vi "Auto Control.vi"   [LabVIEW 2018]
uses:
  <vilib>/Rock Robotics/Network Tables/NT Write String Array.vi
  SubSystems/Drive Train/Drive Train Global.vi
  Robot Global Data.vi
  SubSystems/Hatch Panel Intake/Hatch Panel Intake Global.vi
  SubSystems/Lift/Lift Global.vi
  SubSystems/Cargo Intake/Cargo Intake Global.vi
types:
  T1 = cluster{"X PID":cluster{"proportional gain (Kc)":dbl, "integral time (Ti, min)":dbl, "derivative time (Td, min)":dbl}, "Y PID":cluster{"proportional gain (Kc)":dbl, "integral time (Ti, min)":dbl, "derivative time (Td, min)":dbl}, "Z PID":cluster{"proportional gain (Kc)":dbl, "integral time (Ti, min)":dbl, "derivative time (Td, min)":dbl}}
  T2 = enum16{"Hatch Panel Zone 1", "Hatch Panel Zone 2", "Hatch Panel Zone 3", "Cargo Zone 1", "Cargo Zone 2", "Cargo Zone 3", "Cargo Ship Zone"}
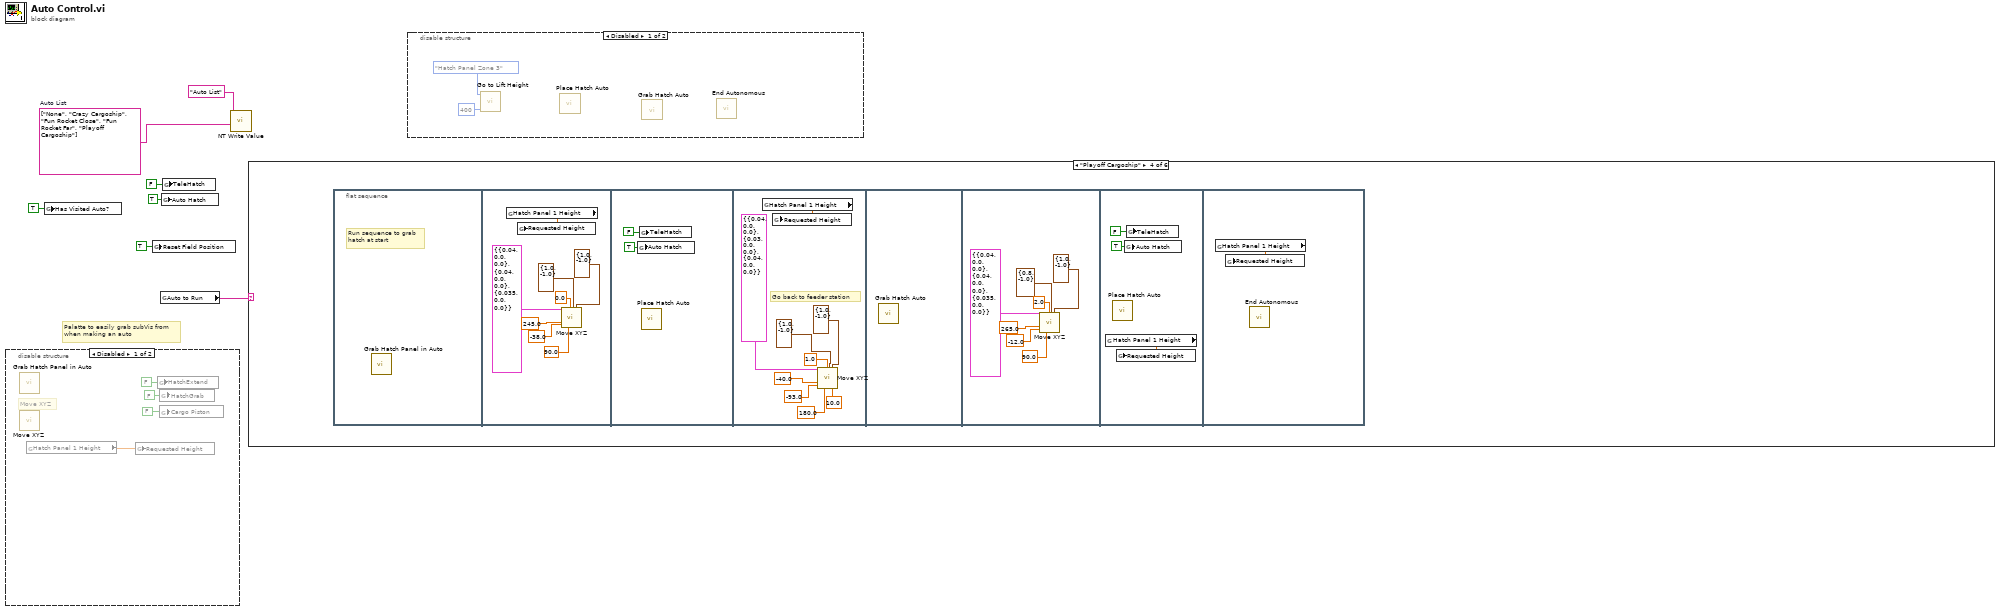
[diagram p0: block diagram]
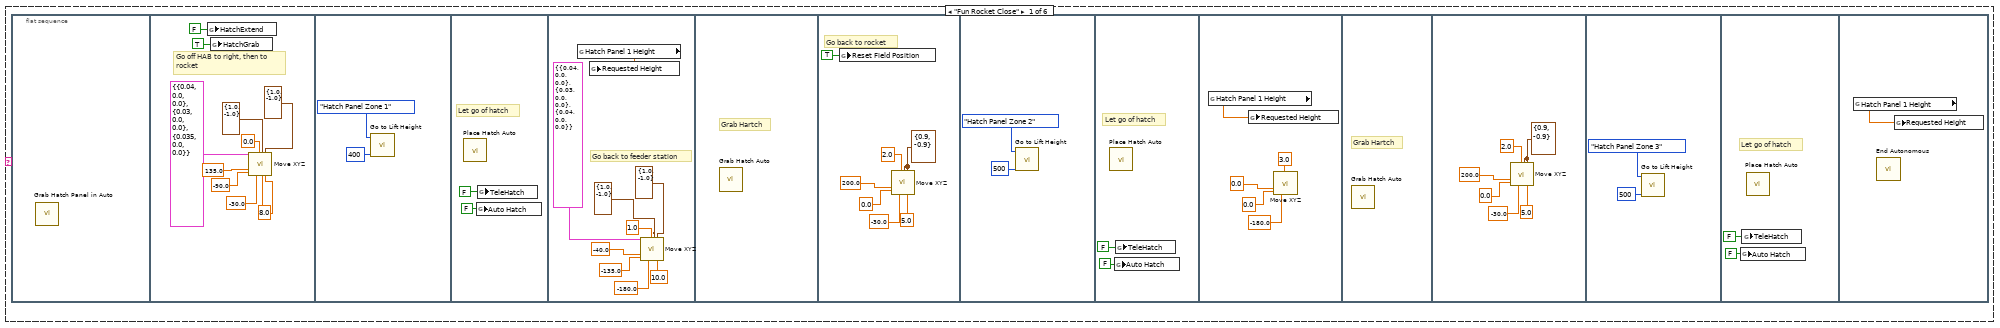
[diagram p4: hidden frame]
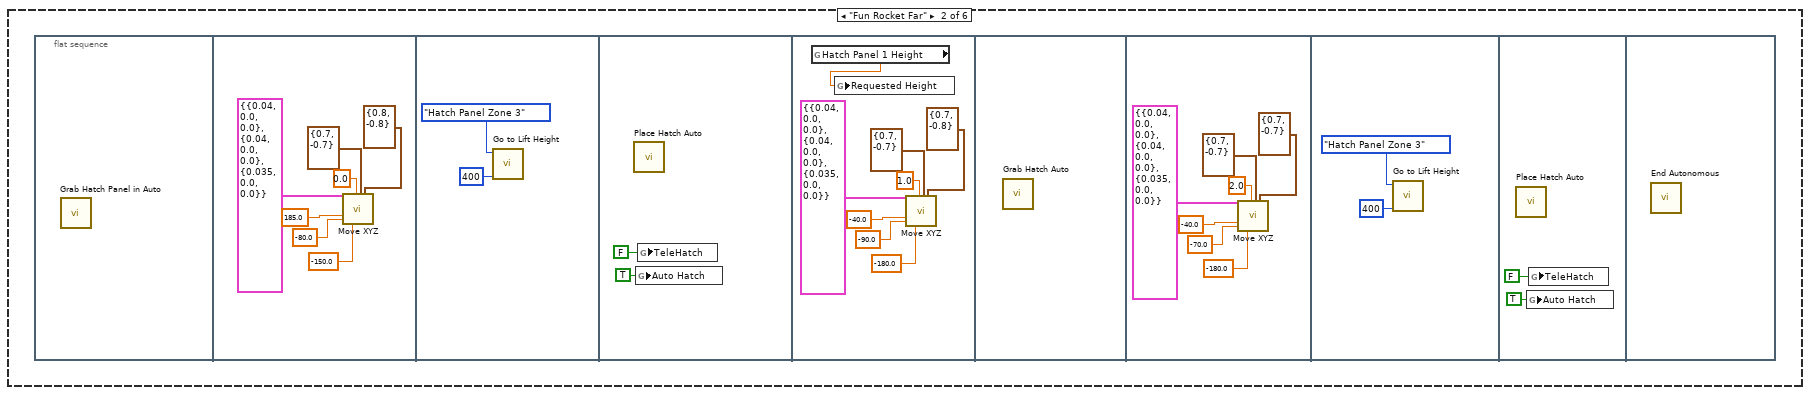
[diagram p5: hidden frame]
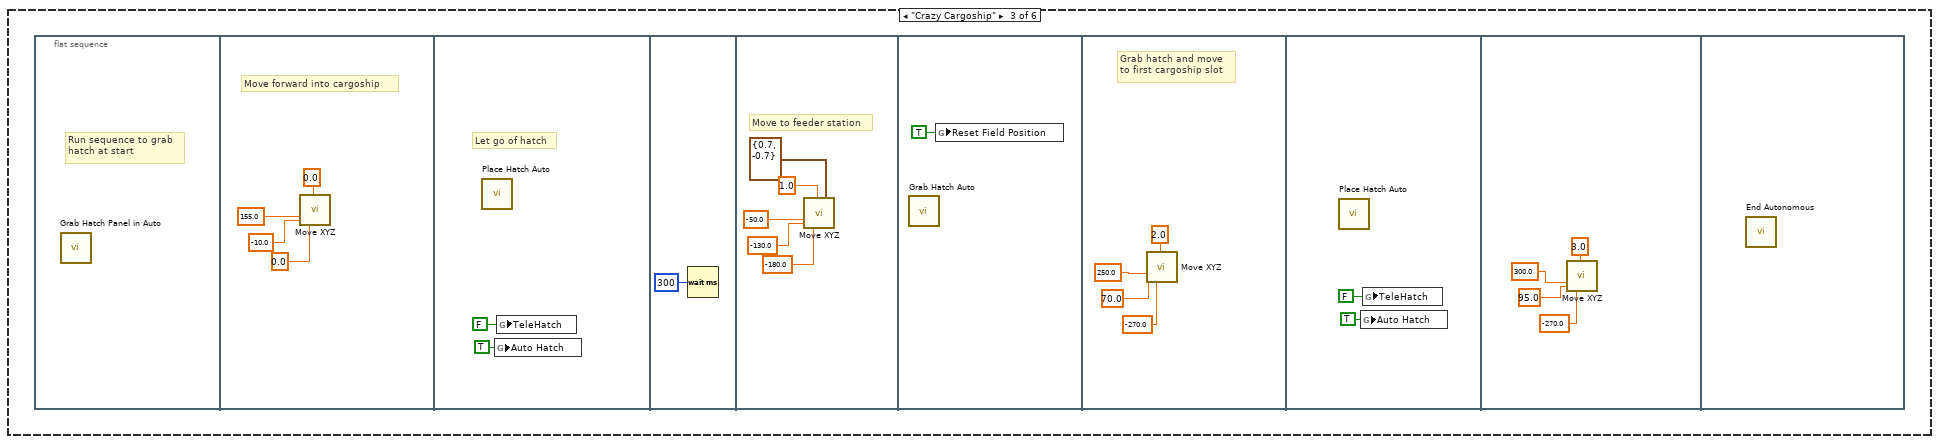
[diagram p6: hidden frame]
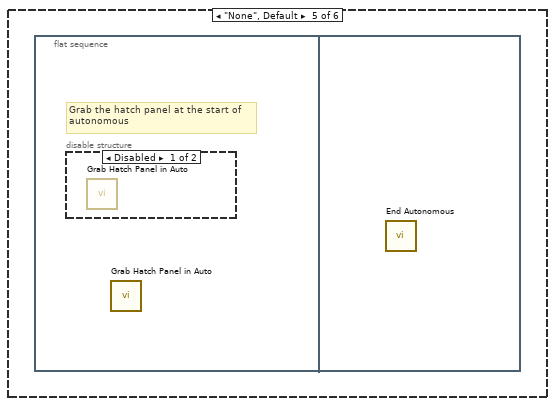
[diagram p7: hidden frame]
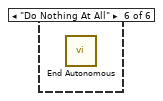
[diagram p9: hidden frame]
diagram:
  w6 = string[] ["None", "Crazy Cargoship", "Fun Rocket Close", "Fun Rocket Far", "Playoff Cargoship"]  # Auto List
  # "Palatte to easily grab subVis from\nwhen making an auto"
  n1 = disable-structure shown="Disabled" {
    frame Disabled {
      # "Move XYZ"
      n2 = call "Move XYZ.vi"() -> ()  [unwired: 28 in]
      n3 = call "Grab Hatch Panel in Auto.vi"() -> ()  [unwired: 12 in]
      n4 = global read "Lift Global.vi" "Hatch Panel 1 Height"() -> (w11:dbl)
      n5 = global write "Lift Global.vi" "Requested Height"(w11) -> ()
      n6 = global write "Hatch Panel Intake Global.vi" "HatchExtend"(FALSE ("HatchExtend")) -> ()
      n7 = global write "Hatch Panel Intake Global.vi" "HatchGrab"(FALSE ("HatchGrab")) -> ()
      n8 = global write "Cargo Intake Global.vi" "Cargo Piston"(FALSE ("Cargo Piston")) -> ()
    }
    frame Enabled {
    }
  }
  n9 = global write "Robot Global Data.vi" "Has Visited Auto?"(TRUE ("Has Visited Auto?")) -> ()
  n10 = global write "Drive Train Global.vi" "Reset Field Position"(TRUE ("Reset Field Position")) -> ()
  n11 = global read "Robot Global Data.vi" "Auto to Run"() -> (w5:string)
  n12 = global write "Hatch Panel Intake Global.vi" "Auto Hatch"(TRUE ("TeleHatch")) -> ()
  n13 = global write "Hatch Panel Intake Global.vi" "TeleHatch"(FALSE ("TeleHatch")) -> ()
  n14 = call-poly <vilib>:"NT Write Value.vi"("String Array"=w6, "Name"="Auto List") -> ()  [unwired: 9 in, 1 out]
  n15 = case shown="\"Playoff Cargoship\"" w5 {
    frame "Fun Rocket Close" {
      n16 = flat-sequence {
        frame #0 {
          n17 = call "Grab Hatch Panel in Auto.vi"() -> ()  [unwired: 12 in]
        }
        frame #1 {
          w15 = 8.0 ("X Stop Threshold")
          # "Go off HAB to right, then to\nrocket"
          n18 = global write "Hatch Panel Intake Global.vi" "HatchExtend"(FALSE ("HatchExtend")) -> ()
          n19 = global write "Hatch Panel Intake Global.vi" "HatchGrab"(TRUE ("HatchGrab")) -> ()
          n20 = call "Move XYZ.vi"("PID Gains In"=T1 {"X PID"={"proportional gain (Kc)"=0.04, "integral time (Ti, min)"=0.0, "derivative time (Td, min)"=0.0}, "Y PID"={"proportional gain (Kc)"=0.03, "integral time (Ti, min)"=0.0, "derivative time (Td, min)"=0.0}, "Z PID"={"proportional gain (Kc)"=0.035, "integral time (Ti, min)"=0.0, "derivative time (Td, min)"=0.0}}, "Y Target"=135.0, "X Target"=-90.0, "Gyro Target"=-30.0, "Movement"=0.0, "X Output Range"=cluster{"output high":dbl, "output low":dbl} {"output high"=1.0, "output low"=-1.0}, "X Stop Threshold"=w15, "Y Output Range"=cluster{"output high":dbl, "output low":dbl} {"output high"=1.0, "output low"=-1.0} ("X Output Range"), "Y Stop Threshold"=w15) -> ()  [unwired: 19 in]
        }
        frame #2 {
          n21 = call "Go to Lift Height.vi"("Time to Settle"=u32 400, "Lift Height to Go To"=T2."Hatch Panel Zone 1" ("y")) -> ()  [unwired: 10 in]
        }
        frame #3 {
          # "Let go of hatch"
          n22 = call "Place Hatch Auto.vi"() -> ()  [unwired: 12 in]
          n23 = global write "Hatch Panel Intake Global.vi" "Auto Hatch"(FALSE ("TeleHatch")) -> ()
          n24 = global write "Hatch Panel Intake Global.vi" "TeleHatch"(FALSE ("TeleHatch")) -> ()
        }
        frame #4 {
          # "Go back to feeder station"
          n25 = global read "Lift Global.vi" "Hatch Panel 1 Height"() -> (w26:dbl)
          n26 = global write "Lift Global.vi" "Requested Height"(w26) -> ()
          n27 = call "Move XYZ.vi"("PID Gains In"=T1 {"X PID"={"proportional gain (Kc)"=0.04, "integral time (Ti, min)"=0.0, "derivative time (Td, min)"=0.0}, "Y PID"={"proportional gain (Kc)"=0.03, "integral time (Ti, min)"=0.0, "derivative time (Td, min)"=0.0}, "Z PID"={"proportional gain (Kc)"=0.04, "integral time (Ti, min)"=0.0, "derivative time (Td, min)"=0.0}}, "Y Target"=-40.0, "X Target"=-135.0, "Gyro Target"=-180.0, "Movement"=1.0, "X Output Range"=cluster{"output high":dbl, "output low":dbl} {"output high"=1.0, "output low"=-1.0}, "Y Output Range"=cluster{"output high":dbl, "output low":dbl} {"output high"=1.0, "output low"=-1.0} ("X Output Range"), "Y Stop Threshold"=10.0) -> ()  [unwired: 20 in]
        }
        frame #5 {
          # "Grab Hartch"
          n28 = call "Grab Hatch Auto.vi"() -> ()  [unwired: 12 in]
        }
        frame #6 {
          w35 = cluster{"output high":dbl, "output low":dbl} {"output high"=0.9, "output low"=-0.9} ("Y Output Range")
          # "Go back to rocket"
          n29 = global write "Drive Train Global.vi" "Reset Field Position"(TRUE ("Reset Field Position")) -> ()
          n30 = call "Move XYZ.vi"("Y Target"=200.0, "X Target"=0.0, "Gyro Target"=-30.0, "Movement"=2.0, "X Output Range"=w35, "Y Output Range"=w35, "Y Stop Threshold"=5.0) -> ()  [unwired: 21 in]
        }
        frame #7 {
          n31 = call "Go to Lift Height.vi"("Time to Settle"=u32 500, "Lift Height to Go To"=T2."Hatch Panel Zone 2" ("y")) -> ()  [unwired: 10 in]
        }
        frame #8 {
          # "Let go of hatch"
          n32 = call "Place Hatch Auto.vi"() -> ()  [unwired: 12 in]
          n33 = global write "Hatch Panel Intake Global.vi" "Auto Hatch"(FALSE ("TeleHatch")) -> ()
          n34 = global write "Hatch Panel Intake Global.vi" "TeleHatch"(FALSE ("TeleHatch")) -> ()
        }
        frame #9 {
          n35 = global read "Lift Global.vi" "Hatch Panel 1 Height"() -> (w50:dbl)
          n36 = global write "Lift Global.vi" "Requested Height"(w50) -> ()
          n37 = call "Move XYZ.vi"("Y Target"=0.0, "X Target"=0.0, "Gyro Target"=-180.0, "Movement"=3.0) -> ()  [unwired: 24 in]
        }
        frame #10 {
          # "Grab Hartch"
          n38 = call "Grab Hatch Auto.vi"() -> ()  [unwired: 12 in]
        }
        frame #11 {
          w51 = cluster{"output high":dbl, "output low":dbl} {"output high"=0.9, "output low"=-0.9} ("Y Output Range")
          n39 = call "Move XYZ.vi"("Y Target"=200.0, "X Target"=0.0, "Gyro Target"=-30.0, "Movement"=2.0, "X Output Range"=w51, "Y Output Range"=w51, "Y Stop Threshold"=5.0) -> ()  [unwired: 21 in]
        }
        frame #12 {
          n40 = call "Go to Lift Height.vi"("Time to Settle"=u32 500, "Lift Height to Go To"=T2."Hatch Panel Zone 3" ("y")) -> ()  [unwired: 10 in]
        }
        frame #13 {
          # "Let go of hatch"
          n41 = global write "Hatch Panel Intake Global.vi" "Auto Hatch"(FALSE ("TeleHatch")) -> ()
          n42 = global write "Hatch Panel Intake Global.vi" "TeleHatch"(FALSE ("TeleHatch")) -> ()
          n43 = call "Place Hatch Auto.vi"() -> ()  [unwired: 12 in]
        }
        frame #14 {
          n44 = global read "Lift Global.vi" "Hatch Panel 1 Height"() -> (w61:dbl)
          n45 = call "End Autonomous.vi"() -> ()  [unwired: 12 in]
          n46 = global write "Lift Global.vi" "Requested Height"(w61) -> ()
        }
      }
    }
    frame "Fun Rocket Far" {
      n47 = flat-sequence {
        frame #0 {
          n48 = call "Grab Hatch Panel in Auto.vi"() -> ()  [unwired: 12 in]
        }
        frame #1 {
          n49 = call "Move XYZ.vi"("PID Gains In"=T1 {"X PID"={"proportional gain (Kc)"=0.04, "integral time (Ti, min)"=0.0, "derivative time (Td, min)"=0.0}, "Y PID"={"proportional gain (Kc)"=0.04, "integral time (Ti, min)"=0.0, "derivative time (Td, min)"=0.0}, "Z PID"={"proportional gain (Kc)"=0.035, "integral time (Ti, min)"=0.0, "derivative time (Td, min)"=0.0}}, "Y Target"=185.0, "X Target"=-80.0, "Gyro Target"=-150.0, "Movement"=0.0, "X Output Range"=cluster{"output high":dbl, "output low":dbl} {"output high"=0.7, "output low"=-0.7}, "Y Output Range"=cluster{"output high":dbl, "output low":dbl} {"output high"=0.8, "output low"=-0.8} ("X Output Range")) -> ()  [unwired: 21 in]
        }
        frame #2 {
          n50 = call "Go to Lift Height.vi"("Time to Settle"=u32 400, "Lift Height to Go To"=T2."Hatch Panel Zone 3" ("y")) -> ()  [unwired: 10 in]
        }
        frame #3 {
          n51 = call "Place Hatch Auto.vi"() -> ()  [unwired: 12 in]
          n52 = global write "Hatch Panel Intake Global.vi" "Auto Hatch"(TRUE ("TeleHatch")) -> ()
          n53 = global write "Hatch Panel Intake Global.vi" "TeleHatch"(FALSE ("TeleHatch")) -> ()
        }
        frame #4 {
          n54 = global read "Lift Global.vi" "Hatch Panel 1 Height"() -> (w73:dbl)
          n55 = global write "Lift Global.vi" "Requested Height"(w73) -> ()
          n56 = call "Move XYZ.vi"("PID Gains In"=T1 {"X PID"={"proportional gain (Kc)"=0.04, "integral time (Ti, min)"=0.0, "derivative time (Td, min)"=0.0}, "Y PID"={"proportional gain (Kc)"=0.04, "integral time (Ti, min)"=0.0, "derivative time (Td, min)"=0.0}, "Z PID"={"proportional gain (Kc)"=0.035, "integral time (Ti, min)"=0.0, "derivative time (Td, min)"=0.0}}, "Y Target"=-40.0, "X Target"=-90.0, "Gyro Target"=-180.0, "Movement"=1.0, "X Output Range"=cluster{"output high":dbl, "output low":dbl} {"output high"=0.7, "output low"=-0.7}, "Y Output Range"=cluster{"output high":dbl, "output low":dbl} {"output high"=0.7, "output low"=-0.8} ("X Output Range")) -> ()  [unwired: 21 in]
        }
        frame #5 {
          n57 = call "Grab Hatch Auto.vi"() -> ()  [unwired: 12 in]
        }
        frame #6 {
          n58 = call "Move XYZ.vi"("PID Gains In"=T1 {"X PID"={"proportional gain (Kc)"=0.04, "integral time (Ti, min)"=0.0, "derivative time (Td, min)"=0.0}, "Y PID"={"proportional gain (Kc)"=0.04, "integral time (Ti, min)"=0.0, "derivative time (Td, min)"=0.0}, "Z PID"={"proportional gain (Kc)"=0.035, "integral time (Ti, min)"=0.0, "derivative time (Td, min)"=0.0}}, "Y Target"=-40.0, "X Target"=-70.0, "Gyro Target"=-180.0, "Movement"=2.0, "X Output Range"=cluster{"output high":dbl, "output low":dbl} {"output high"=0.7, "output low"=-0.7}, "Y Output Range"=cluster{"output high":dbl, "output low":dbl} {"output high"=0.7, "output low"=-0.7} ("X Output Range")) -> ()  [unwired: 21 in]
        }
        frame #7 {
          n59 = call "Go to Lift Height.vi"("Time to Settle"=u32 400, "Lift Height to Go To"=T2."Hatch Panel Zone 3" ("y")) -> ()  [unwired: 10 in]
        }
        frame #8 {
          n60 = call "Place Hatch Auto.vi"() -> ()  [unwired: 12 in]
          n61 = global write "Hatch Panel Intake Global.vi" "Auto Hatch"(TRUE ("TeleHatch")) -> ()
          n62 = global write "Hatch Panel Intake Global.vi" "TeleHatch"(FALSE ("TeleHatch")) -> ()
        }
        frame #9 {
          n63 = call "End Autonomous.vi"() -> ()  [unwired: 12 in]
        }
      }
    }
    frame "Crazy Cargoship" {
      n64 = flat-sequence {
        frame #0 {
          # "Run sequence to grab\nhatch at start"
          n65 = call "Grab Hatch Panel in Auto.vi"() -> ()  [unwired: 12 in]
        }
        frame #1 {
          # "Move forward into cargoship"
          n66 = call "Move XYZ.vi"("Y Target"=155.0, "X Target"=-10.0, "Gyro Target"=0.0, "Movement"=0.0) -> ()  [unwired: 24 in]
        }
        frame #2 {
          # "Let go of hatch"
          n67 = call "Place Hatch Auto.vi"() -> ()  [unwired: 12 in]
          n68 = global write "Hatch Panel Intake Global.vi" "Auto Hatch"(TRUE ("TeleHatch")) -> ()
          n69 = global write "Hatch Panel Intake Global.vi" "TeleHatch"(FALSE ("TeleHatch")) -> ()
        }
        frame #3 {
          n70 = Wait (ms)(milliseconds to wait=u32 300) -> ()  [unwired: 1 out]
        }
        frame #4 {
          # "Move to feeder station"
          n71 = call "Move XYZ.vi"("Y Target"=-50.0, "X Target"=-130.0, "Gyro Target"=-180.0, "Movement"=1.0, "Y Output Range"=cluster{"output high":dbl, "output low":dbl} {"output high"=0.7, "output low"=-0.7}) -> ()  [unwired: 23 in]
        }
        frame #5 {
          n72 = call "Grab Hatch Auto.vi"() -> ()  [unwired: 12 in]
          n73 = global write "Drive Train Global.vi" "Reset Field Position"(TRUE ("Reset Field Position")) -> ()
        }
        frame #6 {
          # "Grab hatch and move\nto first cargoship slot"
          n74 = call "Move XYZ.vi"("Y Target"=250.0, "X Target"=70.0, "Gyro Target"=-270.0, "Movement"=2.0) -> ()  [unwired: 24 in]
        }
        frame #7 {
          n75 = call "Place Hatch Auto.vi"() -> ()  [unwired: 12 in]
          n76 = global write "Hatch Panel Intake Global.vi" "Auto Hatch"(TRUE ("TeleHatch")) -> ()
          n77 = global write "Hatch Panel Intake Global.vi" "TeleHatch"(FALSE ("TeleHatch")) -> ()
        }
        frame #8 {
          n78 = call "Move XYZ.vi"("Y Target"=300.0, "X Target"=95.0, "Gyro Target"=-270.0, "Movement"=3.0) -> ()  [unwired: 24 in]
        }
        frame #9 {
          n79 = call "End Autonomous.vi"() -> ()  [unwired: 12 in]
        }
      }
    }
    frame "Playoff Cargoship" {
      n80 = flat-sequence {
        frame #0 {
          # "Run sequence to grab\nhatch at start"
          n81 = call "Grab Hatch Panel in Auto.vi"() -> ()  [unwired: 12 in]
        }
        frame #1 {
          n82 = global read "Lift Global.vi" "Hatch Panel 1 Height"() -> (w115:dbl)
          n83 = global write "Lift Global.vi" "Requested Height"(w115) -> ()
          n84 = call "Move XYZ.vi"("PID Gains In"=T1 {"X PID"={"proportional gain (Kc)"=0.04, "integral time (Ti, min)"=0.0, "derivative time (Td, min)"=0.0}, "Y PID"={"proportional gain (Kc)"=0.04, "integral time (Ti, min)"=0.0, "derivative time (Td, min)"=0.0}, "Z PID"={"proportional gain (Kc)"=0.035, "integral time (Ti, min)"=0.0, "derivative time (Td, min)"=0.0}}, "Y Target"=245.0, "X Target"=-38.0, "Gyro Target"=90.0, "Movement"=0.0, "X Output Range"=cluster{"output high":dbl, "output low":dbl} {"output high"=1.0, "output low"=-1.0}, "Y Output Range"=cluster{"output high":dbl, "output low":dbl} {"output high"=1.0, "output low"=-1.0} ("X Output Range")) -> ()  [unwired: 21 in]
        }
        frame #2 {
          n85 = global write "Hatch Panel Intake Global.vi" "Auto Hatch"(TRUE ("TeleHatch")) -> ()
          n86 = global write "Hatch Panel Intake Global.vi" "TeleHatch"(FALSE ("TeleHatch")) -> ()
          n87 = call "Place Hatch Auto.vi"() -> ()  [unwired: 12 in]
        }
        frame #3 {
          # "Go back to feeder station"
          n88 = global read "Lift Global.vi" "Hatch Panel 1 Height"() -> (w125:dbl)
          n89 = global write "Lift Global.vi" "Requested Height"(w125) -> ()
          n90 = call "Move XYZ.vi"("PID Gains In"=T1 {"X PID"={"proportional gain (Kc)"=0.04, "integral time (Ti, min)"=0.0, "derivative time (Td, min)"=0.0}, "Y PID"={"proportional gain (Kc)"=0.03, "integral time (Ti, min)"=0.0, "derivative time (Td, min)"=0.0}, "Z PID"={"proportional gain (Kc)"=0.04, "integral time (Ti, min)"=0.0, "derivative time (Td, min)"=0.0}}, "Y Target"=-40.0, "X Target"=-93.0, "Gyro Target"=180.0, "Movement"=1.0, "X Output Range"=cluster{"output high":dbl, "output low":dbl} {"output high"=1.0, "output low"=-1.0}, "Y Output Range"=cluster{"output high":dbl, "output low":dbl} {"output high"=1.0, "output low"=-1.0} ("X Output Range"), "Y Stop Threshold"=10.0) -> ()  [unwired: 20 in]
        }
        frame #4 {
          n91 = call "Grab Hatch Auto.vi"() -> ()  [unwired: 12 in]
        }
        frame #5 {
          n92 = call "Move XYZ.vi"("PID Gains In"=T1 {"X PID"={"proportional gain (Kc)"=0.04, "integral time (Ti, min)"=0.0, "derivative time (Td, min)"=0.0}, "Y PID"={"proportional gain (Kc)"=0.04, "integral time (Ti, min)"=0.0, "derivative time (Td, min)"=0.0}, "Z PID"={"proportional gain (Kc)"=0.035, "integral time (Ti, min)"=0.0, "derivative time (Td, min)"=0.0}}, "Y Target"=265.0, "X Target"=-12.0, "Gyro Target"=90.0, "Movement"=2.0, "X Output Range"=cluster{"output high":dbl, "output low":dbl} {"output high"=0.8, "output low"=-1.0}, "Y Output Range"=cluster{"output high":dbl, "output low":dbl} {"output high"=1.0, "output low"=-1.0} ("X Output Range")) -> ()  [unwired: 21 in]
        }
        frame #6 {
          n93 = global read "Lift Global.vi" "Hatch Panel 1 Height"() -> (w143:dbl)
          n94 = call "Place Hatch Auto.vi"() -> ()  [unwired: 12 in]
          n95 = global write "Lift Global.vi" "Requested Height"(w143) -> ()
          n96 = global write "Hatch Panel Intake Global.vi" "Auto Hatch"(TRUE ("TeleHatch")) -> ()
          n97 = global write "Hatch Panel Intake Global.vi" "TeleHatch"(FALSE ("TeleHatch")) -> ()
        }
        frame #7 {
          n98 = global read "Lift Global.vi" "Hatch Panel 1 Height"() -> (w144:dbl)
          n99 = global write "Lift Global.vi" "Requested Height"(w144) -> ()
          n100 = call "End Autonomous.vi"() -> ()  [unwired: 12 in]
        }
      }
    }
    frame "None", Default {
      n101 = flat-sequence {
        frame #0 {
          # "Grab the hatch panel at the start of \nautonomous"
          n102 = disable-structure shown="Disabled" {
            frame Disabled {
              n103 = call "Grab Hatch Panel in Auto.vi"() -> ()  [unwired: 12 in]
            }
            frame Enabled {
            }
          }
          n104 = call "Grab Hatch Panel in Auto.vi"() -> ()  [unwired: 12 in]
        }
        frame #1 {
          n105 = call "End Autonomous.vi"() -> ()  [unwired: 12 in]
        }
      }
    }
    frame "Do Nothing At All" {
      n106 = call "End Autonomous.vi"() -> ()  [unwired: 12 in]
    }
  }
  n107 = disable-structure shown="Disabled" {
    frame Disabled {
      n108 = call "Go to Lift Height.vi"("Time to Settle"=u32 400, "Lift Height to Go To"=T2."Hatch Panel Zone 3" ("y")) -> ()  [unwired: 10 in]
      n109 = call "Place Hatch Auto.vi"() -> ()  [unwired: 12 in]
      n110 = call "Grab Hatch Auto.vi"() -> ()  [unwired: 12 in]
      n111 = call "End Autonomous.vi"() -> ()  [unwired: 12 in]
    }
    frame Enabled {
    }
  }
